vi "PROB ATTEN SETTING.vi"(8 "ATTENUATIONs:":T1(radio), 10 "CHANNEL":enum32{"CH 1", "CH 2", "CH 3", "CH 4"}(radio), 11 "VISA resource name 2":refnum<visa-resource-name>="GPIB0::1::INSTR") -> ()   [LabVIEW 2018]
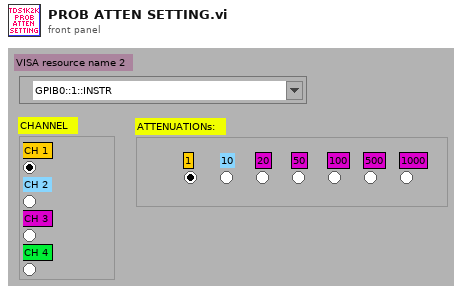
[diagram p1: front panel]
types:
  T1 = enum32{"1", "10", "20", "50", "100", "500", "1000"}
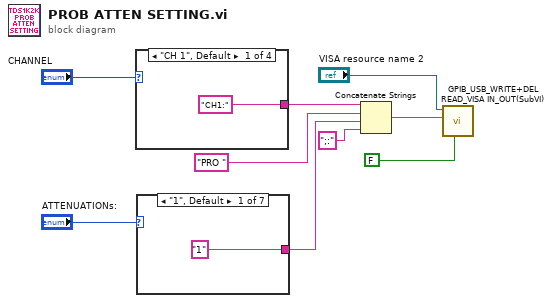
[diagram p0: block diagram]
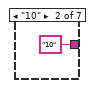
[diagram p2: hidden frame]
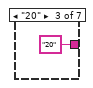
[diagram p3: hidden frame]
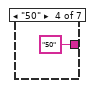
[diagram p4: hidden frame]
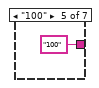
[diagram p5: hidden frame]
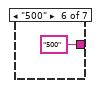
[diagram p6: hidden frame]
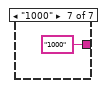
[diagram p7: hidden frame]
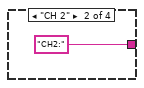
[diagram p8: hidden frame]
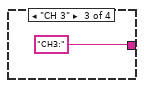
[diagram p9: hidden frame]
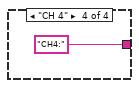
[diagram p10: hidden frame]
diagram:
  n1 = case shown="\"CH 1\", Default" "CHANNEL" {
    tunnel: ["CH1:" "CH2:" "CH3:" "CH4:"] -> w5
    frame "CH 1", Default {
    }
    frame "CH 2" {
    }
    frame "CH 3" {
    }
    frame "CH 4" {
    }
  }
  n2 = case shown="\"1\", Default" "ATTENUATIONs:" {
    tunnel: ["1" "10" "20" "50" "100" "500" "1000"] -> w8
    frame "1", Default {
    }
    frame "10" {
    }
    frame "20" {
    }
    frame "50" {
    }
    frame "100" {
    }
    frame "500" {
    }
    frame "1000" {
    }
  }
  n3 = Concatenate Strings(w5, "PRO ", w8, ";:") -> (w2:string)
  n4 = call "GPIB_USB_WRITE+DEL READ_VISA IN_OUT(SubVI).vi"("VISA resource IN"="VISA resource name 2", "GPIB/USB WRITE"=w2, 4:FALSE ("READ GPIB")) -> ()  [unwired: 3 in, 3 out]
